vi "Read Sub Panel MSG.vi"(8 "error in (no error)":errorcluster, 11 "MENSAJE in":refnum<class "MENSAJE.lvclass">) -> (0 "error out":errorcluster, 2 "Sub Panel MSG":refnum<vi>, 3 "MENSAJE out":refnum<class "MENSAJE.lvclass">)   [LabVIEW 2020, in "MENSAJE.lvlib" / "MENSAJE.lvclass"]
uses:
  MENSAJE.lvclass
  MENSAJE.lvclass/MENSAJE.ctl
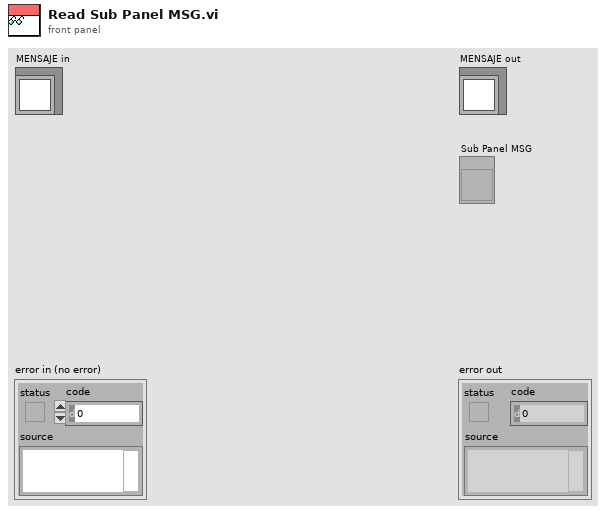
[diagram p1: front panel]
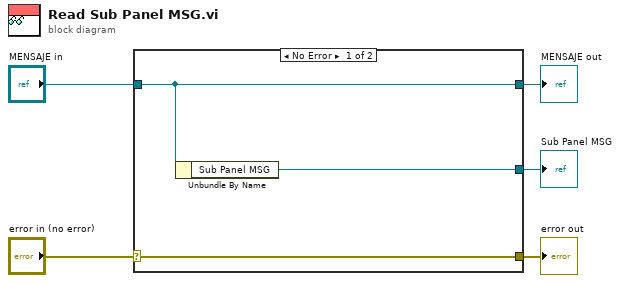
[diagram p0: block diagram]
diagram:
  n1 = case shown="No Error" "error in (no error)" {
    selector: "error in (no error)" -> [w8 w9]
    tunnel: [w8 w9] -> w4
    tunnel: [w7 w10] -> w2
    tunnel: "MENSAJE in" -> [w7 w10]
    tunnel: [w6 _] -> w1
    frame No Error {
      n2 = Unbundle By Name(w7) -> ("Sub Panel MSG"=w6:refnum<vi>)
    }
    frame Error {
    }
  }
  "error out" <- w4
  "MENSAJE out" <- w2
  "Sub Panel MSG" <- w1
